vi "example-rx-c-api.vi"() -> ()   [LabVIEW 2024]
uses:
  <vilib>/Analysis/2dsp.llb/Complex FFT.vi
  uhd (generated from wizard into user.lib - manually fixed for rx example)/uhd.lvlib
  <vilib>/Analysis/NI_AALPro.lvlib
panel:
  out "output cluster":cluster{dbl, dbl, dbl[]}(graph)
  in  "drop initial samples":i32=20000
  in  "ant":string="RX2"
  out "ant_out out":string="RX2"
  out "Waveform Graph":sgl[][](graph)
  out "items_recvd (sum)":u64=1020000
  out "error out":errorcluster
  out "items_recvd":u64=2040
  in  "num_samps":u64=1000000
  out "freq_out out":dbl=1000000000.0 format="%#_6p"
  in  "target_freq":dbl=1000000000.0 format="%#_6p"
  out "gain_out out":dbl
  in  "gain":dbl
  out "rate_out out":dbl=1000000.0 format="%#_6p"
  in  "chan":u64
  in  "rate":dbl=1000000.0 format="%#_6p"
  in  "args":string="type=b200"
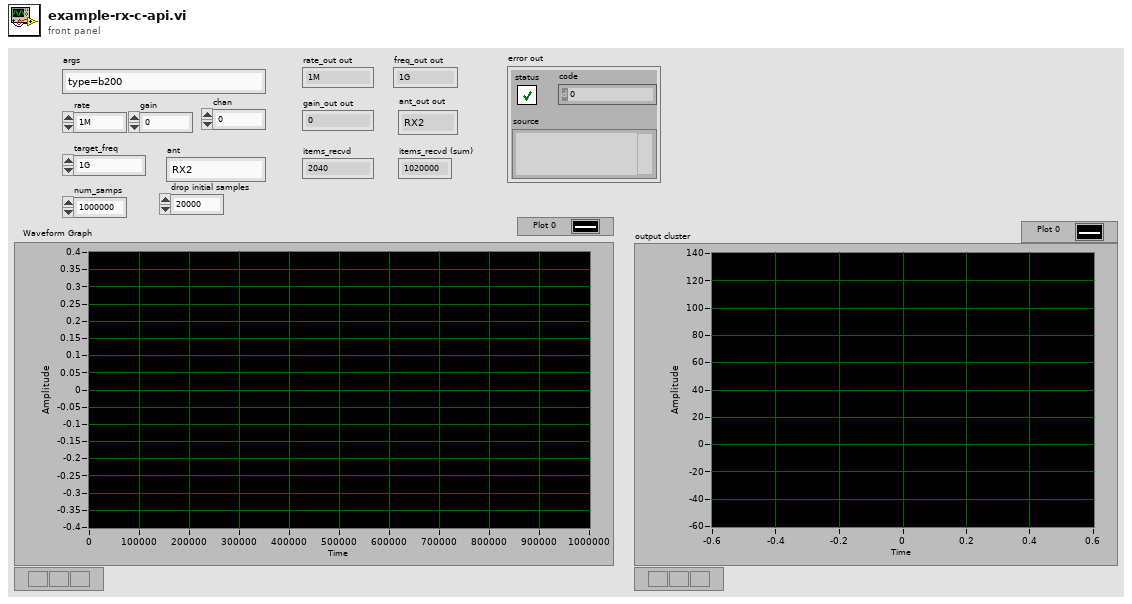
[diagram p1: front panel]
types:
  T1 = cluster{"stream_mode":u32, "@dummy control@":i8, "@dummy control@":i8, "@dummy control@":i8, "@dummy control@":i8, "num_samps":u64, "stream_now":i32, "@dummy control@":i8, "@dummy control@":i8, "@dummy control@":i8, "@dummy control@":i8, "time_spec_full_secs":i64, "time_spec_frac_secs":dbl}
  T2 = cluster{"cpu_format":string, "otw_format":string, "args":string, "channel_list":u64[], "n_channels":i32}
  T3 = cluster{"target_freq":dbl, "rf_freq_policy":u32, "@dummy control@":i8, "@dummy control@":i8, "@dummy control@":i8, "@dummy control@":i8, "rf_freq":dbl, "dsp_freq_policy":u32, "@dummy control@":i8, "@dummy control@":i8, "@dummy control@":i8, "@dummy control@":i8, "dsp_freq":dbl, "args":u64}
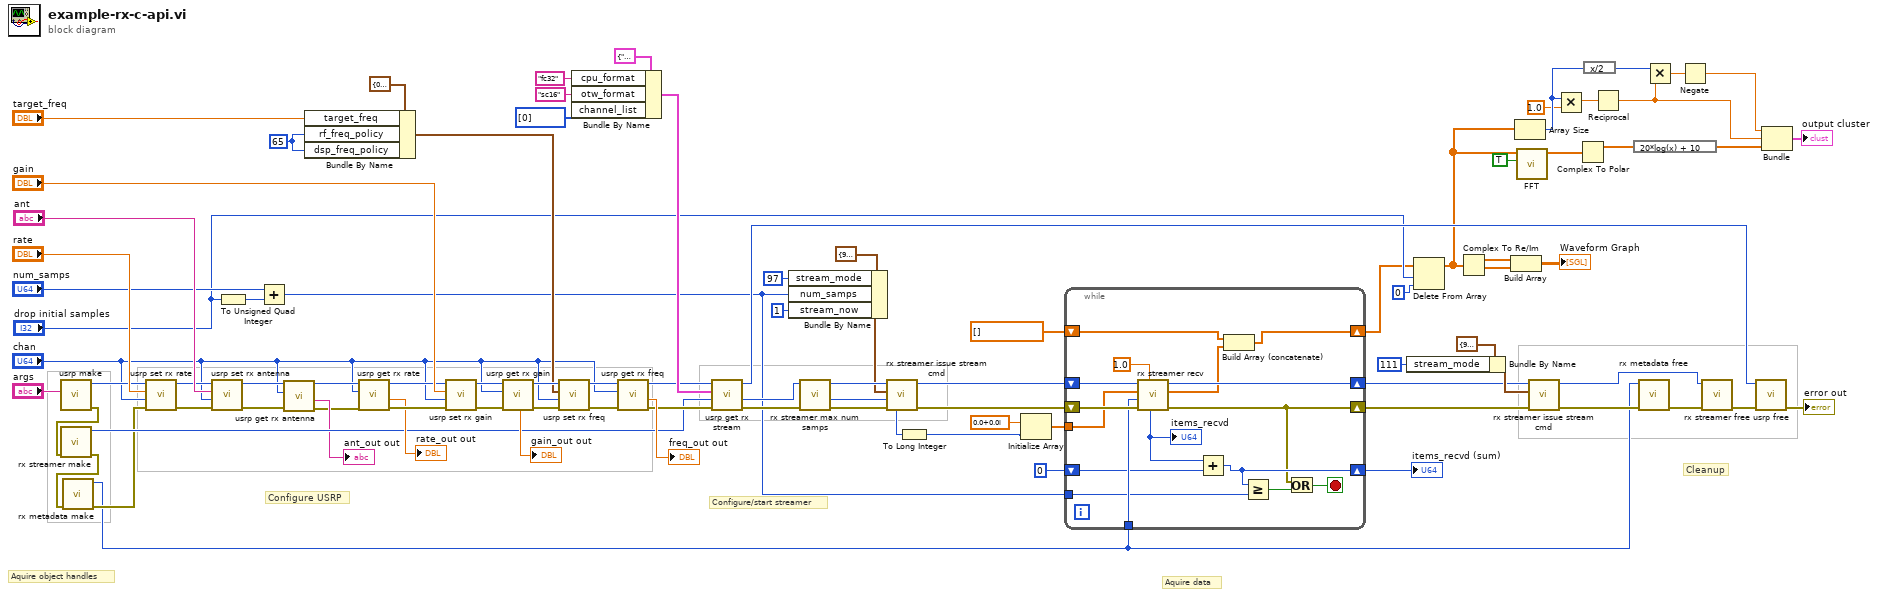
[diagram p0: block diagram]
diagram:
  w74 = u32 65 ("rf_freq_policy")
  # "Cleanup"
  # "Aquire data"
  # "Configure/start streamer"
  # "Configure USRP"
  # "Aquire object handles"
  n1 = call "usrp make.vi"("args"="args") -> ("error out"=w88:errorcluster, "h"=w49:u64)  [unwired: 8 in, 1 out]
  n2 = call "rx streamer make.vi"("error in (no error)"=w88) -> ("error out"=w87:errorcluster, "h 3"=w46:u64)  [unwired: 8 in, 1 out]
  n3 = call "rx metadata make.vi"("error in (no error)"=w87) -> ("error out"=w23:errorcluster, "handle out"=w14:u64)  [unwired: 8 in, 1 out]
  n4 = call "usrp set rx rate.vi"("error in (no error)"=w23, "chan"="chan", "rate"="rate", "h"=w49) -> ("error out"=w35:errorcluster, "h 2"=w39:u64)  [unwired: 5 in, 1 out]
  n5 = call "usrp set rx antenna.vi"("error in (no error)"=w35, "chan"="chan", "ant"="ant", "h"=w39) -> ("error out"=w37:errorcluster, "h 2"=w38:u64)  [unwired: 5 in, 1 out]
  n6 = To Unsigned Quad Integer(1:"drop initial samples") -> (0:w27:u64)
  n7 = Add(x="num_samps", y=w27) -> (x+y=w28:u64)
  n8 = call "usrp get rx antenna.vi"("error in (no error)"=w37, "chan"="chan", "h"=w38) -> ("error out"=w34:errorcluster, "ant_out out"=→"ant_out out":string)  [unwired: 5 in, 2 out]
  n9 = Bundle By Name(cluster=T3 {"target_freq"=0.0, "rf_freq_policy"=65, "@dummy control@"=0, "@dummy control@"=0, "@dummy control@"=0, "@dummy control@"=0, "rf_freq"=0.0, "dsp_freq_policy"=65, "@dummy control@"=0, "@dummy control@"=0, "@dummy control@"=0, "@dummy control@"=0, "dsp_freq"=0.0, "args"=0} ("tune_request"), "target_freq"="target_freq", "rf_freq_policy"=w74, "dsp_freq_policy"=w74) -> (w73:T3)
  n10 = call "usrp get rx rate.vi"("error in (no error)"=w34, "chan"="chan", "h"=w39) -> ("error out"=w85:errorcluster, "rate_out out"=→"rate_out out":dbl, "h 2"=w80:u64)  [unwired: 5 in, 1 out]
  n11 = call "usrp set rx gain.vi"("error in (no error)"=w85, "chan"="chan", "gain"="gain", "h"=w80) -> ("error out"=w82:errorcluster, "h 2"=w81:u64)  [unwired: 5 in, 1 out]
  n12 = call "usrp get rx gain.vi"("error in (no error)"=w82, "chan"="chan", "h"=w81) -> ("error out"=w77:errorcluster, "h 2"=w78:u64, "gain_out out"=→"gain_out out":dbl)  [unwired: 5 in, 1 out]
  n13 = call "usrp set rx freq.vi"("error in (no error)"=w77, "chan"="chan", "tune_request"=w73, "h"=w78) -> ("error out"=w71:errorcluster, "h 3"=w72:u64)  [unwired: 2 in, 4 out]
  n14 = Bundle By Name(cluster=T2 {"cpu_format"="", "otw_format"="", "args"="", "channel_list"=[], "n_channels"=0} ("stream_args"), "cpu_format"="fc32", "otw_format"="sc16", "channel_list"=u64[] [0]) -> (w64:T2)
  n15 = call "usrp get rx freq.vi"("error in (no error)"=w71, "chan"="chan", "h"=w72) -> ("error out"=w69:errorcluster, "freq_out out"=→"freq_out out":dbl, "h 2"=w47:u64)  [unwired: 5 in, 1 out]
  n16 = call "usrp get rx stream.vi"("error in (no error)"=w69, "h 3"=w46, "stream_args"=w64, "h"=w47) -> ("error out"=w63:errorcluster, "h 4"=w48:u64, "h 2"=w50:u64)  [unwired: 3 in, 2 out]
  n17 = Bundle By Name(cluster=T1 {"stream_mode"=97, "@dummy control@"=0, "@dummy control@"=0, "@dummy control@"=0, "@dummy control@"=0, "num_samps"=0, "stream_now"=0, "@dummy control@"=0, "@dummy control@"=0, "@dummy control@"=0, "@dummy control@"=0, "time_spec_full_secs"=0, "time_spec_frac_secs"=0.0} ("stream_cmd"), "stream_mode"=u32 97, "num_samps"=w28, "stream_now"=1) -> (w58:T1)
  n18 = call "rx streamer max num samps.vi"("error in (no error)"=w63, "h"=w48) -> ("error out"=w61:errorcluster, "max_num_samps_out out"=w45:u64, "h 2"=w62:u64)  [unwired: 6 in, 1 out]
  n19 = call "rx streamer issue stream cmd.vi"("error in (no error)"=w61, "stream_cmd"=w58, "h"=w62) -> ("error out"=w22:errorcluster, "h 2"=w57:u64)  [unwired: 6 in, 1 out]
  n20 = To Long Integer(number=w45) -> (32bit integer=w32:i32)
  n21 = Initialize Array(csg 0.0+0.0i ("single precision complex"), w32) -> (w30:csg[])
  n22 = while {
    tunnel: w14 -> [w104]
    tunnel: w30 -> [w103]
    shift-right: [w92] -> w21
    shift-left: w22 -> [w105]
    shift-right: [w100] -> w53
    shift-left: w57 -> [w102]
    shift-right: [w97] -> w41
    shift-left: u64 0 ("items_recvd out") -> [w98]
    tunnel: w28 -> [w96]
    shift-right: [w93] -> w25
    shift-left: csg[] [] ("buffs out") -> [w95]
    stop <- w90 stop-if-true
    n23 = call "rx streamer recv.vi"("timeout"=1.0, "error in (no error)"=w105, "md"=w104, "buffs"=w103, "h"=w102) -> ("error out"=w92:errorcluster, "buffs out"=w94:csg[], "h 2"=w100:u64, "items_recvd out"=w99:u64)  [unwired: 1 in, 2 out]
    "items_recvd" <- w99
    n24 = Add(x=w99, y=w98) -> (x+y=w97:u64)
    n25 = Build Array (concatenate)(w95, w94) -> (w93:csg[])
    n26 = Greater Or Equal?(x=w97, y=w96) -> (x >= y?=w91:bool)
    n27 = Or(x=w92, y=w91) -> (x .or. y?=w90:bool)
  }
  "items_recvd (sum)" <- w41
  n28 = Bundle By Name(cluster=T1 {"stream_mode"=97, "@dummy control@"=0, "@dummy control@"=0, "@dummy control@"=0, "@dummy control@"=0, "num_samps"=0, "stream_now"=0, "@dummy control@"=0, "@dummy control@"=0, "@dummy control@"=0, "@dummy control@"=0, "time_spec_full_secs"=0, "time_spec_frac_secs"=0.0} ("stream_cmd"), "stream_mode"=u32 111) -> (w54:T1)
  n29 = Delete From Array(array=w25, length="drop initial samples", index=0) -> (array with subset deleted=w12:csg[])  [unwired: 1 out]
  n30 = Complex To Re/Im(x + iy=w12) -> (x=w19:sgl[], y=w20:sgl[])
  n31 = Build Array(w19, w20) -> (→"Waveform Graph":sgl[][])
  n32 = Array Size(array=w12) -> (size(s)=w8:i32)
  n33 = call-poly <vilib>:"FFT.vi"("shift?"=TRUE, "X"=w12) -> ("FFT {X}"=w11:cdb[])  [unwired: 8 in, 1 out]
  n34 = call "rx streamer issue stream cmd.vi"("error in (no error)"=w21, "stream_cmd"=w54, "h"=w53) -> ("error out"=w52:errorcluster, "h 2"=w51:u64)  [unwired: 6 in, 1 out]
  n35 = Multiply(x=w8, y=1.0) -> (x*y=w6:dbl)
  n36 = Complex To Polar(r * e^(i*theta)=w11) -> (r=w10:dbl[])  [unwired: 1 out]
  n37 = expression code="x/2"(w8) -> (w5:i32)
  n38 = Reciprocal(x=w6) -> (1/x=w2:dbl)
  n39 = expression code="20*log(x) + 10"(w10) -> (w9:dbl[])
  n40 = call "rx metadata free.vi"("error in (no error)"=w52, "handle"=w14) -> ("error out"=w17:errorcluster)  [unwired: 7 in, 2 out]
  n41 = Multiply(x=w5, y=w2) -> (x*y=w4:dbl)
  n42 = Negate(x=w4) -> (-x=w3:dbl)
  n43 = call "rx streamer free.vi"("error in (no error)"=w17, "h"=w51) -> ("error out"=w16:errorcluster)  [unwired: 7 in, 2 out]
  n44 = call "usrp free.vi"("error in (no error)"=w16, "h"=w50) -> ("error out"=→"error out":errorcluster)  [unwired: 7 in, 2 out]
  n45 = Bundle(w3, w2, w9) -> (→"output cluster":cluster{dbl, dbl, dbl[]})  [unwired: 1 in]
